vi "Gradient2Fringe.vi"(9 "freq (Hz)":dbl=1589645.882716435, 10 "erot(V/cm)":dbl=22.0, 11 "dB(mG/cm)":dbl=40.0) -> (3 "Frequency(Hz)":dbl)   [LabVIEW 2012]
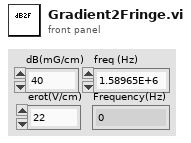
[diagram p1: front panel]
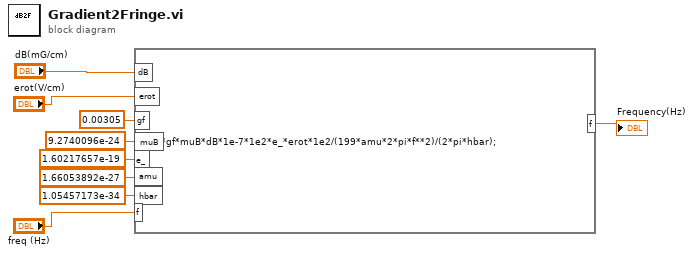
[diagram p0: block diagram]
diagram:
  n1 = formula code="f=3*gf*muB*dB*1e-7*1e2*e_*erot*1e2/(199*amu*2*pi*f**2)/(2*pi*hbar);"("dB"="dB(mG/cm)", "erot"="erot(V/cm)", "gf"=0.00305 ("input variable"), "muB"=9.2740096e-24 ("input variable"), "e_"=1.60217657e-19 ("input variable"), "amu"=1.66053892e-27 ("input variable"), "hbar"=1.05457173e-34 ("input variable"), "f"="freq (Hz)") -> ("f"=→"Frequency(Hz)":dbl)
